vi "HFRR ADV v016 new software.vi"() -> ()   [LabVIEW 2025] (continued)
                    n4032 = call <vilib>:"System Exec.vi"("run minimized? (F)"=TRUE, "wait until completion? (T)"=TRUE, "working directory"=path "C:/LAB-IQ-NXT", "command line"="C:\\LAB-IQ-NXT\\JPost.bat") -> ("standard error"=→"Respose From Server":string, "standard output"=w5132:string)  [unwired: 4 in, 2 out]
                    "standard output" <- w5132
                    n4033 = Match Pattern(string=w5132, regular expression="JSON Check String") -> (match substring=w5130:string, offset past match=w5129:i32)  [unwired: 1 in, 2 out]
                    n4034 = Equal?(x=w5130, y="JSON Check String") -> (x = y?=→"Upload \nConfirmed":bool)
                  }
                }
              }
            }
            n4035 = local read "Quit"() -> (w5053:bool)
          }
        }
      }
    }
    frame Enabled {
    }
  }
  n4036 = disable-structure shown="Disabled" {
    disable-tunnel: _ -> [w5215 _]
    frame Disabled {
      n4037 = while {
        shift-right: [w5223] -> w5211
        shift-left: _ -> [w5224]
        shift-right: [w5221] -> w5212
        shift-left: errorcluster {"status"=TRUE, "code"=0, "source"="Init"} ("error out") -> [w5222]
        shift-right: [w5219] -> _
        shift-left: "" -> [w5220]
        tunnel: [w5217] -> _
        tunnel: w5215 -> [_]
        i -> [w5217]
        stop <- w5216 stop-if-true
        n4038 = flat-sequence {
          tunnel: [w5225] -> w5218
          frame #0 {
            n4039 = Wait (ms)(milliseconds to wait=10.0 ("Delay")) -> (millisecond timer value=w5225:u32)
          }
        }
        n4040 = case shown="No Error" w5222 {
          selector: w5222 -> [w5255 w5374]
          tunnel: [w5238 w5376] -> w5223
          tunnel: [w5237 w5375] -> w5221
          tunnel: w5224 -> [w5256 w5368]
          tunnel: w5220 -> [w5236 w5367]
          tunnel: [w5235 w5367] -> w5219
          tunnel: w5218 -> [_ _]
          frame No Error {
            n4041 = Concatenate Strings("\r", "\n") -> (w5247:string)  [unwired: 1 in]
            n4042 = case shown="True" w5248 {
              tunnel: w5256 -> [w5280 w5287]
              tunnel: w5255 -> [w5279 w5286]
              tunnel: [w5280 w5285] -> w5254
              tunnel: [w5279 w5284] -> w5234
              tunnel: w5247 -> [_ w5283]
              frame False {
              }
              frame True {
                n4043 = VISA Write(VISA resource name=w5287, write buffer=w5283, error in (no error)=w5286) -> (VISA resource name out=w5285:refnum<visa-resource-name>, error out=w5284:errorcluster)  [unwired: 1 out]
                n4044 = local write "Read String"("") -> ()
                n4045 = local write item#-1(FALSE) -> ()
              }
            }
            n4046 = property class="Instr"(reference=w5254, error in=w5234) -> (reference out=w5253:refnum<visa-resource-name>, error out=w5252:errorcluster, "Serial Settings:Number of Bytes at Serial Port"=w5251:u32)
            n4047 = Greater?(x=w5251, y=u32 100) -> (0:w5249:bool)
            n4048 = case shown="True" w5249 {
              tunnel: w5253 -> [w5290 w5314]
              tunnel: w5252 -> [w5289 w5313]
              tunnel: w5251 -> [_ w5312]
              tunnel: [w5290 w5311] -> w5240
              tunnel: [w5289 w5310] -> w5239
              tunnel: w5236 -> [w5288 w5309]
              tunnel: [w5288 ""] -> w5235
              frame False {
              }
              frame True {
                w5299 = u32 6 ("y")
                # "Page 84 of \nmanual"
                n4049 = VISA Read(VISA resource name=w5314, byte count=w5312, error in (no error)=w5313) -> (VISA resource name out=w5311:refnum<visa-resource-name>, read buffer=w5307:string, error out=w5310:errorcluster)  [unwired: 1 out]
                n4050 = while {
                  tunnel: w5307 -> [w5363]
                  tunnel: [w5359] -> w5301 mode=indexing
                  tunnel: [w5353] -> w5305 mode=indexing
                  tunnel: [w5351] -> _
                  i -> [w5351]
                  stop <- w5356 stop-if-true
                  n4051 = String Subset(string=w5363, offset (0)=w5351) -> (substring=w5358:string)  [unwired: 1 in]
                  n4052 = String To Byte Array(string=w5358) -> (unsigned byte array=w5362:u8[])
                  n4053 = String Length(string=w5358) -> (length=w5357:i32)
                  n4054 = Index Array(array=w5362) -> (element=w5361:u8)  [unwired: 1 in]
                  n4055 = Equal To 0?(x=w5357) -> (x = 0?=w5356:bool)
                  n4056 = Number To Boolean Array(number=w5361) -> (Boolean array=w5355:bool[])
                  n4057 = Reverse 1D Array(array=w5355) -> (reversed array=w5354:bool[])
                  n4058 = And(x=w5355, y=bool[] [FALSE, FALSE, FALSE, FALSE, FALSE, FALSE, TRUE, TRUE] ("Boolean array")) -> (x .and. y?=w5359:bool[])
                  n4059 = And(x=w5354, y=bool[] [FALSE, FALSE, TRUE, TRUE, TRUE, TRUE, TRUE, TRUE] ("Boolean array")) -> (x .and. y?=w5353:bool[])
                }
                n4060 = Concatenate Strings(w5309, w5307) -> (→"Read String":string)
                n4061 = while {
                  tunnel: w5301 -> [w5350] mode=indexing
                  tunnel: [w5346] -> w5304
                  i -> [w5346]
                  stop <- w5347 stop-if-true
                  n4062 = Search 1D Array(1D array=w5350, element=TRUE) -> (index of element=w5348:i32)  [unwired: 1 in]
                  n4063 = Less Than 0?(x=w5348) -> (x < 0?=w5347:bool)
                }
                n4064 = Delete From Array(array=w5305, length=w5304, index (row)=0) -> (array with subset deleted=w5300:bool[][])  [unwired: 1 in, 1 out]
                n4065 = Array Size(array=w5300) -> (size(s)=w5302:i32[])
                n4066 = Index Array(array=w5302) -> (element=w5294:i32)  [unwired: 1 in]
                n4067 = Greater?(x=w5294, y=w5299) -> (0:w5297:bool)
                n4068 = Subtract(x=w5294, y=w5299) -> (x-y=w5298:u32)
                n4069 = Select(t=w5298, s=w5297, f=u32 0) -> (s? t:f=w5295:u32)
                n4070 = while {
                  tunnel: w5300 -> [w5333]
                  tunnel: [w5335] -> w5293 mode=indexing
                  tunnel: w5295 -> [w5317]
                  i -> [w5334]
                  stop <- w5332 stop-if-true
                  w5324 = 6 ("index")
                  w5323 = 2 ("length")
                  # "Page 65 of \nmanual"
                  n4071 = Multiply(x=u32 3 ("y"), y=w5334) -> (x*y=w5331:u32)
                  n4072 = Divide(x=u32 102 ("y"), y=u32 65520) -> (x/y=w5341:dbl)
                  n4073 = Greater Or Equal?(x=w5331, y=w5317) -> (x >= y?=w5332:bool)
                  n4074 = Index Array(array=w5333, index (row) #1=w5331) -> (element #1=w5329:bool[], element #2=w5328:bool[], element #3=w5327:bool[])  [unwired: 5 in]
                  n4075 = Reverse 1D Array(array=w5329) -> (reversed array=w5322:bool[])
                  n4076 = Reverse 1D Array(array=w5328) -> (reversed array=w5326:bool[])
                  n4077 = Reverse 1D Array(array=w5327) -> (reversed array=w5325:bool[])
                  n4078 = Delete From Array(array=w5322, length=w5323, index=w5324) -> (array with subset deleted=w5318:bool[])  [unwired: 1 out]
                  n4079 = Delete From Array(array=w5326, length=w5323, index=w5324) -> (array with subset deleted=w5319:bool[])  [unwired: 1 out]
                  n4080 = Delete From Array(array=w5325, length=w5323, index=w5324) -> (array with subset deleted=w5320:bool[])  [unwired: 1 out]
                  n4081 = Insert Into Array(array=bool[] [] ("Boolean array"), new element #1=w5318, new element #2=w5319, new element #3=w5320) -> (w5321:bool[])  [unwired: 1 in]
                  n4082 = Boolean Array To Number(Boolean array=w5321) -> (number=w5330:u32)
                  n4083 = Multiply(x=w5341, y=w5330) -> (x*y=w5340:dbl)
                  n4084 = Decrement(x=w5340) -> (x-1=w5339:dbl)
                  n4085 = Divide(x=w5339, y=u32 100) -> (x/y=w5337:dbl)
                  n4086 = Multiply(x=w5337, y=u32 10) -> (x*y=w5335:dbl)
                }
                n4087 = Delete From Array(array=w5293) -> (array with subset deleted=w5292:dbl[])  [unwired: 2 in, 1 out]
                "Waveform Graph 5" <- w5292
                "Waveform Chart 3" <- w5292
                n4088 = call-poly <vilib>:"Mean.vi"("X"=w5292) -> ("mean"=w5291:dbl)  [unwired: 1 out]
                n4089 = case shown="True" {
                  selector: _ -> [_ _]
                  tunnel: w5291 -> [_ w5316]
                  frame False {
                  }
                  frame True {
                    n4090 = local write item#-1(FALSE ("Zero 4")) -> ()
                    "z_measure" <- w5316
                  }
                }
              }
            }
            n4091 = local read item#-1() -> (w5231)
            n4092 = local read item#-1() -> (w5230)
            n4093 = local read item#-1() -> (w5232)
            n4094 = local read item#-1() -> (w5229)
            n4095 = case shown="True" w5227 {
              tunnel: w5231 -> [_ w5259]
              tunnel: w5232 -> [_ w5258]
              frame False {
              }
              frame True {
                n4096 = Build Array(w5259, w5258) -> (w5257:void[])
                n4097 = local read item#-1() -> (w5262)
                n4098 = Build Array (concatenate)(w5262, w5257) -> (w5260:void[])
                n4099 = local write item#-1(w5260) -> ()
                n4100 = local write item#-1(FALSE ("Boolean 8")) -> ()
              }
            }
            n4101 = call "Build XY Graph"("Enable"=w5229, "Reset"=w5230, "Y Input"=w5232, "X Input"=w5231) -> ("XY Graph"=w5228:cluster{"Y":dbl[], "Y":dbl[]}[])  [unwired: 6 in, 1 out]
            n4102 = case shown="True" {
              selector: _ -> [_ _]
              frame False {
              }
              frame True {
                n4103 = local read item#-1() -> (w5263)
                n4104 = Index Array(array=w5263, index (col) #1=0 ("disabled index (col)"), index (col) #2=1 ("index (col)")) -> (element #1=w5265, element #2=w5264)  [unwired: 2 in]
                n4105 = call <vilib>:"Linear Fit.vi"("Y"=w5265, "X"=w5264) -> ()  [unwired: 9 in, 5 out]
                n4106 = local write item#-1(FALSE ("Boolean 9")) -> ()
              }
            }
            n4107 = case shown="True" {
              selector: _ -> [_ _]
              frame False {
              }
              frame True {
                n4108 = local write item#-1(dbl[][] [] ("Captured Values")) -> ()
                n4109 = local write item#-1(FALSE ("Boolean 7")) -> ()
              }
            }
            n4110 = Concatenate Strings("\r", "\n") -> (w5242:string, w5241:string)
            n4111 = case shown="True" w5233 {
              tunnel: w5240 -> [w5272 w5278]
              tunnel: w5239 -> [w5271 w5277]
              tunnel: [w5272 w5276] -> w5238
              tunnel: [w5271 w5275] -> w5237
              tunnel: w5242 -> [_ w5274]
              frame False {
              }
              frame True {
                n4112 = VISA Write(VISA resource name=w5278, write buffer=w5274, error in (no error)=w5277) -> (VISA resource name out=w5276:refnum<visa-resource-name>, error out=w5275:errorcluster)  [unwired: 1 out]
                n4113 = local write item#-1(FALSE ("WRITE")) -> ()
              }
            }
          }
          frame Error {
            w5366 = u16 10 items=["1.0"=10, "1.5"=15, "2.0"=20] ("stop bits (10: 1 bit)")
            n4114 = Wait (ms)(milliseconds to wait=u32 20) -> ()  [unwired: 1 out]
            n4115 = VISA Close(VISA resource name=w5368, error in (no error)=w5374) -> (error out=w5373:errorcluster)
            n4116 = call <vilib>:"Clear Errors.vi"("error in (no error)"=w5373) -> ("error out"=w5372:errorcluster)  [unwired: 5 in, 1 out]
            n4117 = call-poly "VISA Configure Serial Port"("timeout (10sec)"=u32 200, "Enable Termination\nChar (T)"=TRUE ("Enable Termination\nChar (T)"), "baud rate (9600)"=u32 921600, "error in (no error)"=w5372, "stop bits (10: 1 bit)"=w5366) -> ("VISA resource name"=w5364:refnum<visa-resource-name>, "VISA resource name out"=w5376:refnum<visa-resource-name>, "error out"=w5375:errorcluster)  [unwired: 8 in]
          }
        }
        n4118 = local read "Quit"() -> (w5216:bool)
      }
      n4119 = VISA Close(VISA resource name=w5211, error in (no error)=w5212) -> (error out=w5210:errorcluster)
      n4120 = call <vilib>:"Clear Errors.vi"("error in (no error)"=w5210) -> ()  [unwired: 5 in, 2 out]
    }
    frame Enabled {
    }
  }
  n4121 = disable-structure shown="Disabled" {
    disable-tunnel: _ -> [w5381 _]
    frame Disabled {
      n4122 = while {
        tunnel: [w5388] -> _
        shift-right: [w5385] -> w5378
        shift-left: _ -> [w5387]
        shift-right: [w5386] -> w5379
        shift-left: errorcluster {"status"=TRUE, "code"=0, "source"="Init"} ("error out") -> [w5384]
        tunnel: w5381 -> [_]
        i -> [w5388]
        stop <- w5382 stop-if-true
        n4123 = flat-sequence {
          tunnel: w5384 -> [w5479]
          tunnel: [w5479] -> w5383
          frame #0 {
            n4124 = Wait (ms)(milliseconds to wait=u32 50) -> ()  [unwired: 1 out]
          }
        }
        n4125 = case shown="No Error" w5383 {
          selector: w5383 -> [w5429 w5472]
          tunnel: w5387 -> [w5428 w5471]
          tunnel: [w5395 w5462] -> w5386
          tunnel: [w5396 w5470] -> w5385
          frame No Error {
            w5422 = T33 {"Mode"=enum."RTU", "Slave Address"=1} ("Serial Parameters")
            n4126 = call-poly <vilib>:"MB Serial Master Query (poly).vi"("VISA resource name"=w5428, "Starting Address"=i16 1000, "Quantity"=u16 1, "Timeout"=u32 1000, "error in"=w5429, "Serial Parameters"=w5422) -> ("VISA resource name out"=w5423:refnum<visa-resource-name>, "Input Registers"=w5425:u16[], "error out"=w5421:errorcluster)  [unwired: 10 in, 1 out]
            n4127 = Random Number (0-1)() -> (number: 0 to 1=w5410:dbl)
            n4128 = Index Array(array=w5425, index=0) -> (element=w5420:u16)
            n4129 = Subtract(x=w5410, y=0.5) -> (x-y=w5409:dbl)
            n4130 = Divide(x=w5420, y=10 ("index")) -> (x/y=w5414:dbl)
            n4131 = Multiply(x=w5409, y=0.5) -> (x*y=w5408:dbl)
            n4132 = Add(x=w5414, y=w5408) -> (x+y=w5413:dbl)
            n4133 = local read "Amb temp"() -> (w5397:dbl)
            n4134 = Multiply(x=w5413, y=0.2) -> (x*y=w5417:dbl)
            n4135 = Multiply(x=w5397, y=0.8) -> (x*y=w5415:dbl)
            n4136 = Add(x=w5417, y=w5415) -> (x+y=w5398:dbl)
            n4137 = local read "set temp old"() -> (w5392:dbl)
            n4138 = local write "Amb temp"(w5398) -> ()
            n4139 = Select(t="SetTemp 2", s="Heater", f=100.0) -> (s? t:f=w5393:dbl)
            n4140 = Not Equal?(x=w5393, y=w5392) -> (x != y?=w5391:bool)
            n4141 = case shown="True" w5391 {
              tunnel: w5423 -> [w5457 w5459]
              tunnel: [w5456 w5459] -> w5403
              tunnel: w5421 -> [w5455 w5458]
              tunnel: [w5454 w5458] -> w5401
              tunnel: w5393 -> [w5449 _]
              tunnel: w5422 -> [w5451 w5460]
              tunnel: [w5451 w5460] -> w5404
              frame True {
                n4142 = Multiply(x=w5449, y=10 ("index")) -> (x*y=w5448:dbl)
                n4143 = call-poly <vilib>:"MB Serial Master Query (poly).vi"("VISA resource name"=w5457, "Address"=u16 0, "Holding Register"=w5448, "Timeout"=u32 1000, "error in"=w5455, "Serial Parameters"=w5451) -> ("VISA resource name out"=w5456:refnum<visa-resource-name>, "error out"=w5454:errorcluster)  [unwired: 11 in, 1 out]
                "set temp old" <- w5449
              }
              frame False {
              }
            }
            n4144 = flat-sequence {
              tunnel: [w5430] -> _
              tunnel: [w5430] -> w5400
              tunnel: w5401 -> [w5430]
              frame #0 {
                n4145 = Wait (ms)(milliseconds to wait=u32 100) -> ()  [unwired: 1 out]
              }
            }
            n4146 = call "Elapsed Time12"("Time Target (s)"=2.0, "Auto Reset"=TRUE) -> ("Time has Elapsed"=w5405:bool)  [unwired: 10 in, 7 out]
            n4147 = case shown="True" w5405 {
              tunnel: w5404 -> [w5434 w5447]
              tunnel: [w5434 w5447] -> _
              tunnel: [w5433 w5445] -> w5396
              tunnel: w5403 -> [w5433 w5446]
              tunnel: [w5432 w5443] -> w5395
              tunnel: w5400 -> [w5432 w5444]
              frame False {
              }
              frame True {
                n4148 = call-poly <vilib>:"MB Serial Master Query (poly).vi"("VISA resource name"=w5446, "Starting Address"=i16 1003 ("Addr"), "Quantity"=u16 1, "Timeout"=u32 1000, "error in"=w5444, "Serial Parameters"=w5447) -> ("VISA resource name out"=w5445:refnum<visa-resource-name>, "Input Registers"=w5440:u16[], "error out"=w5443:errorcluster)  [unwired: 10 in, 1 out]
                n4149 = Index Array(array=w5440, index=0) -> (element=w5439:u16)
                n4150 = Divide(x=w5439, y=u16 10) -> (x/y=w5435:dbl)
                n4151 = local write "set temp old"(w5435) -> ()
                n4152 = local write "SetTemp"(w5435) -> ()
              }
            }
            "Error Code" <- w5395
            n4153 = Unbundle(w5395) -> ("status"=→"TK4 status":bool)  [unwired: 2 out]
            "SetTemp" <- "SetTemp 2"
          }
          frame Error {
            w5474 = u16 0 items=["None", "Odd", "Even", "Mark", "Space"] ("Parity")
            w5475 = u16 0 items=["None", "XON/XOFF", "RTS/CTS", "XON/XOFF & RTS/CTS", "DTR/DSR", "XON/XOFF & DTR/DSR"] ("Flow Control")
            n4154 = VISA Clear(VISA resource name=w5471, error in (no error)=w5472) -> (VISA resource name out=w5465:refnum<visa-resource-name>, error out=w5463:errorcluster)
            n4155 = VISA Close(VISA resource name=w5465, error in (no error)=w5463) -> (error out=w5464:errorcluster)
            n4156 = call <vilib>:"Clear Errors.vi"("error in (no error)"=w5464) -> ("error out"=w5473:errorcluster)  [unwired: 5 in, 1 out]
            n4157 = Unbundle By Name(T33 {"Mode"=enum."RTU", "Slave Address"=1} ("input cluster")) -> ("Mode"=w5476:enum16{"RTU", "ASCII"})
            n4158 = call <vilib>:"MB Serial Init.vi"("Timeout"=u32 100, "Flow Control"=w5475, "Mode"=w5476, "error in (no error)"=w5473, "Parity"=w5474, "Baud Rate"=u32 9600, "VISA resource name"="Lubrication System COM Port :") -> ("error out"=w5462:errorcluster, "VISA resource name out"=w5470:refnum<visa-resource-name>)  [unwired: 3 in]
            n4159 = local write "set temp old"(0.0 ("set temp old")) -> ()
            n4160 = Unbundle(w5462) -> ("status"=w5461:bool)  [unwired: 2 out]
            n4161 = case shown="True" w5461 {
              selector: w5461 -> [_ w5478]
              frame False {
              }
              frame True {
                n4162 = local write "TK4 status"(w5478) -> ()
              }
            }
          }
        }
        n4163 = local read "Quit"() -> (w5382:bool)
      }
      n4164 = VISA Close(VISA resource name=w5378, error in (no error)=w5379) -> (error out=w5377:errorcluster)
      n4165 = call <vilib>:"Clear Errors.vi"("error in (no error)"=w5377) -> ()  [unwired: 5 in, 2 out]
    }
    frame Enabled {
    }
  }
